vi "tek_Fetch Waveform.vi"(8 "error in (no error)":errorcluster, 9 "Timeout (10000 ms)":u32=10000, 10 "Source (0: Channel 1)":u16(ring) items=["Channel 1", "Channel 2", "Channel 3", "Channel 4", "Math", "Reference A", "Reference B", "Reference C", "Reference D", "FFT"], 11 "VISA resource name":refnum<visa-resource-name>) -> (0 "error out":errorcluster, 1 "Y":dbl[](array[numeric]), 2 "Waveform Data":waveform(dbl)(graph), 3 "VISA resource name out":refnum<visa-resource-name>, 4 "t0":dbl, 5 "dt":dbl)   [LabVIEW 2013, in "Tektronix TDS 200 1000 2000 Series.lvlib"]
doc: "Returns the waveform the oscilloscope acquired for the specified channel. The waveform is from an acquisition that you initiate prior to calling this VI.\n\nYou use the Initiate VI to start an acquisition on the channels that you enable with the Configure Channel VI. The oscilloscope acquires waveforms for the enabled channels concurrently. You must call this VI separately for each enabled channel to obtain the waveforms.\n\nYou can call the Read Waveforms VI instead of using low-level VIs.\n\n<B>Note:</B> Use this VI only with other low-level VIs. The high-level VIs automatically incorporate this functionality. This VI does not check the instrument status."
uses:
  <instrlib>/Tektronix TDS 200 1000 2000 Series/Tektronix TDS 200 1000 2000 Series.lvlib
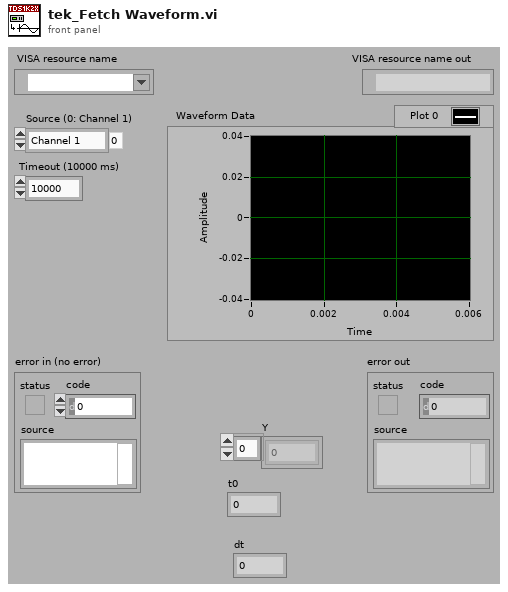
[diagram p1: front panel]
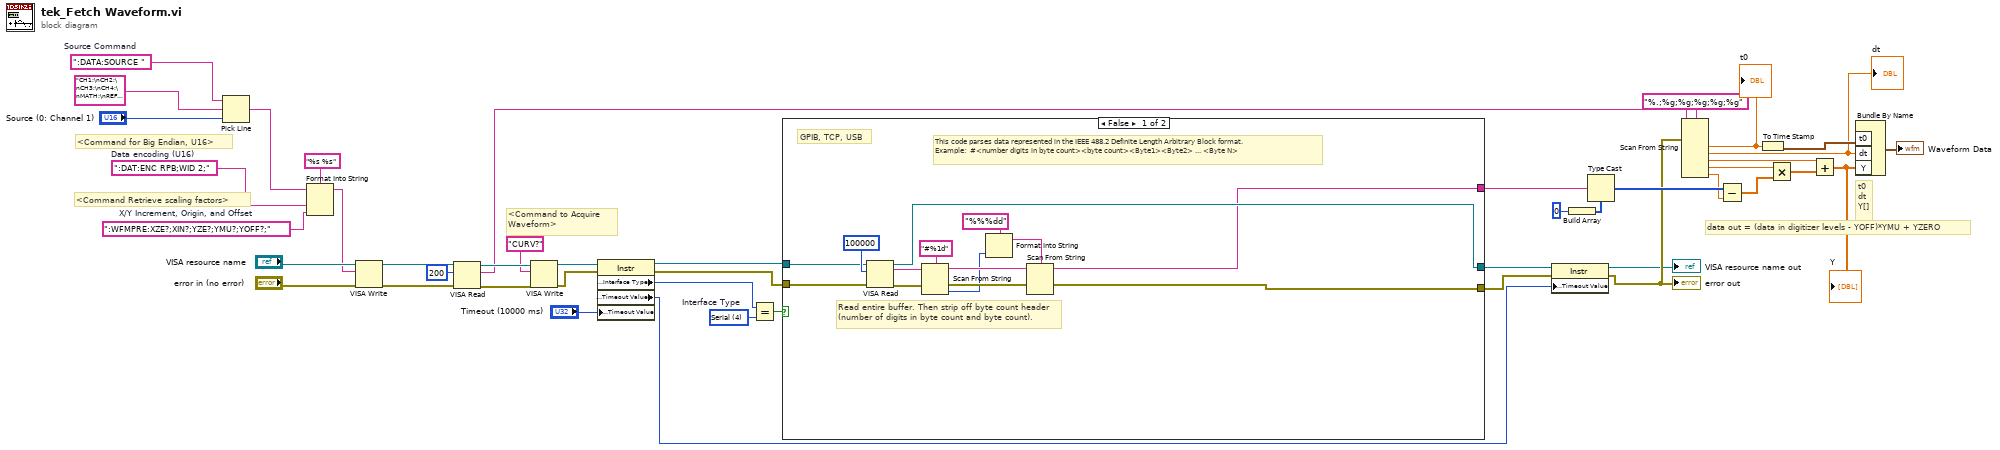
[diagram p0: block diagram]
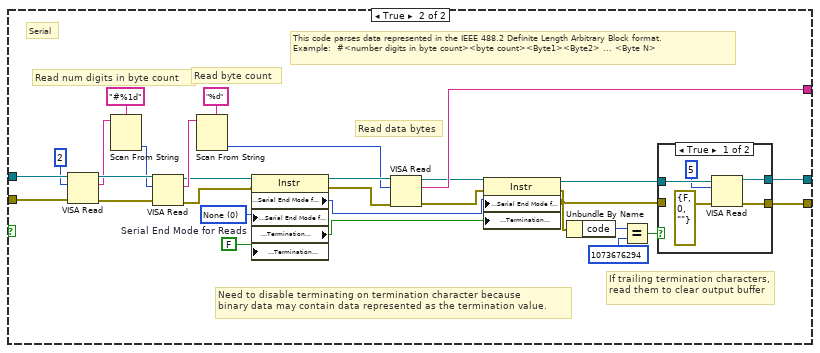
[diagram p2: hidden frame]
diagram:
  w20 = u16 4 items=["GPIB"=1, "VXI"=2, "GPIB-VXI"=3, "Serial"=4, "PXI"=5, "TCPIP"=6, "USB"=7]  # Interface Type
  w29 = ":DATA:SOURCE "  # Source Command
  w26 = ":DAT:ENC RPB;WID 2;"  # Data encoding (U16)
  w27 = ":WFMPRE:XZE?;XIN?;YZE?;YMU?;YOFF?;"  # X/Y Increment, Origin, and Offset
  # "data out = (data in digitizer levels - YOFF)*YMU + YZERO"
  # "<Command to Acquire\nWaveform>"
  # "<Command Retrieve scaling factors>"
  # "<Command for Big Endian, U16>"
  # "t0\ndt\nY[]"
  n1 = Pick Line(string ("")=w29, multi-line string="CH1;\nCH2;\nCH3;\nCH4;\nMATH;\nREFA;\nREFB;\nREFC;\nREFD;\nFFT;", line index="Source (0: Channel 1)") -> (output string=w7:string)
  n2 = Format Into String(format string="%s %s", initial string=w7, w26, w27) -> (resulting string=w25:string)  [unwired: 1 in, 1 out]
  n3 = VISA Write(VISA resource name="VISA resource name", write buffer=w25, error in (no error)="error in (no error)") -> (VISA resource name out=w45:refnum<visa-resource-name>, error out=w44:errorcluster)  [unwired: 1 out]
  n4 = VISA Read(VISA resource name=w45, byte count=u32 200, error in (no error)=w44) -> (VISA resource name out=w42:refnum<visa-resource-name>, read buffer=w35:string, error out=w41:errorcluster)  [unwired: 1 out]
  n5 = VISA Write(VISA resource name=w42, write buffer="CURV?", error in (no error)=w41) -> (VISA resource name out=w11:refnum<visa-resource-name>, error out=w19:errorcluster)  [unwired: 1 out]
  n6 = property class="Instr"(reference=w11, error in=w19, "General Settings:Timeout Value"="Timeout (10000 ms)") -> (reference out=w10:refnum<visa-resource-name>, error out=w18:errorcluster, "Interface Information:Interface Type"=w21:u16, "General Settings:Timeout Value"=w12:u32)
  n7 = Equal?(x=w21, y=w20) -> (x = y?=w17:bool)
  n8 = case shown="False" w17 {
    tunnel: w10 -> [w50 w88]
    tunnel: w18 -> [w49 w87]
    tunnel: [w47 w76] -> w15
    tunnel: [w48 w75] -> w16
    tunnel: [w46 w74] -> w24
    frame False {
      # "Read entire buffer. Then strip off byte count header (number of digits in byte count and byte count)."
      # "This code parses data represented in the IEEE 488.2 Definite Length Arbitrary Block format.\nExample:  #<number digits in byte count><byte count><Byte1><Byte2> ... <Byte N>"
      # "GPIB, TCP, USB"
      n9 = VISA Read(VISA resource name=w50, byte count=u32 100000, error in (no error)=w49) -> (VISA resource name out=w48:refnum<visa-resource-name>, read buffer=w53:string, error out=w51:errorcluster)  [unwired: 1 out]
      n10 = Scan From String(format string="#%1d", input string=w53, error in=w51) -> (remaining string=w57:string, error out=w55:errorcluster, output 1=w54:i32)  [unwired: 2 in, 1 out]
      n11 = Format Into String(format string="%%%dd", w54) -> (resulting string=w56:string)  [unwired: 2 in, 1 out]
      n12 = Scan From String(format string=w56, input string=w57, error in=w55) -> (remaining string=w46:string, error out=w47:errorcluster)  [unwired: 3 in, 1 out]
    }
    frame True {
      w65 = u16 0 items=["None", "Last Bit", "TermChar"]  # Serial End Mode for Reads
      # "Read data bytes"
      # "Read num digits in byte count"
      # "Read byte count"
      # "This code parses data represented in the IEEE 488.2 Definite Length Arbitrary Block format.\nExample:  #<number digits in byte count><byte count><Byte1><Byte2> ... <Byte N>"
      # "Need to disable terminating on termination character because\nbinary data may contain data represented as the termination value."
      # "Serial"
      # "If trailing termination characters, read them to clear output buffer"
      n13 = VISA Read(VISA resource name=w88, byte count=u32 2, error in (no error)=w87) -> (VISA resource name out=w83:refnum<visa-resource-name>, read buffer=w73:string, error out=w84:errorcluster)  [unwired: 1 out]
      n14 = Scan From String(format string="#%1d", input string=w73) -> (output 1=w82:i32)  [unwired: 3 in, 3 out]
      n15 = VISA Read(VISA resource name=w83, byte count=w82, error in (no error)=w84) -> (VISA resource name out=w63:refnum<visa-resource-name>, read buffer=w81:string, error out=w62:errorcluster)  [unwired: 1 out]
      n16 = Scan From String(format string="%d", input string=w81) -> (output 1=w64:i32)  [unwired: 3 in, 3 out]
      n17 = property class="Instr"(reference=w63, error in=w62, "Serial Settings:Serial End Mode for Reads"=w65, "Message Based Settings:Termination Character Enable"=FALSE) -> (reference out=w69:refnum<visa-resource-name>, error out=w70:errorcluster, "Serial Settings:Serial End Mode for Reads"=w68:u16, "Message Based Settings:Termination Character Enable"=w61:bool)
      n18 = VISA Read(VISA resource name=w69, byte count=w64, error in (no error)=w70) -> (VISA resource name out=w67:refnum<visa-resource-name>, read buffer=w74:string, error out=w66:errorcluster)  [unwired: 1 out]
      n19 = property class="Instr"(reference=w67, error in=w66, "Serial Settings:Serial End Mode for Reads"=w68, "Message Based Settings:Termination Character Enable"=w61) -> (reference out=w72:refnum<visa-resource-name>, error out=w71:errorcluster)
      n20 = Unbundle By Name(w71) -> ("code"=w79:i32)
      n21 = Equal?(x=w79, y=1073676294 ("code")) -> (x = y?=w77:bool)
      n22 = case shown="True" w77 {
        tunnel: w72 -> [w93 w95]
        tunnel: w71 -> [_ w94]
        tunnel: [w91 w95] -> w75
        tunnel: [w90 w94] -> w76
        frame True {
          n23 = VISA Read(VISA resource name=w93, byte count=u32 5, error in (no error)=errorcluster {"status"=FALSE, "code"=0, "source"=""}) -> (VISA resource name out=w91:refnum<visa-resource-name>, error out=w90:errorcluster)  [unwired: 2 out]
        }
        frame False {
        }
      }
    }
  }
  n24 = property class="Instr"(reference=w16, error in=w15, "General Settings:Timeout Value"=w12) -> (reference out=→"VISA resource name out":refnum<visa-resource-name>, error out=w14:errorcluster)
  "error out" <- w14
  n25 = Build Array(u16 0) -> (w34:u16[])
  n26 = Type Cast(type=w34, x=w24) -> (*(type *) &x=w36:u16[])
  n27 = Scan From String(format string="%.;%g;%g;%g;%g;%g", input string=w35, error in=w14) -> (output 1=w39:dbl, output 2=w1:dbl, output 3=w2:dbl, output 4=w5:dbl, output 5=w6:dbl)  [unwired: 6 in, 3 out]
  "dt" <- w1
  "t0" <- w39
  n28 = Subtract(x=w36, y=w6) -> (x-y=w37:dbl[])
  n29 = To Time Stamp(1:w39) -> (0:w38:timestamp)
  n30 = Multiply(x=w5, y=w37) -> (x*y=w3:dbl[])
  n31 = Add(x=w2, y=w3) -> (x+y=w4:dbl[])
  "Y" <- w4
  n32 = Bundle By Name("t0"=w38, "dt"=w1, "Y"=w4) -> (→"Waveform Data":waveform(dbl))  [unwired: 1 in]
